vi "wrapandcutimage.vi"(0 "rasterscanned array":sgl[](array[numeric])) -> (1 "imagearray":sgl[][](array[numeric]), 2 "wrap":i32)   [LabVIEW 2015]
panel:
  out "P":dbl
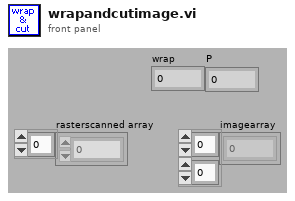
[diagram p1: front panel]
types:
  T1 = typedef "LVRectTypeDef.ctl" = cluster{"Left":i16, "Top":i16, "Right":i16, "Bottom":i16}
  T2 = cluster{"Xpixels":i32, "Vxminref":dbl, "Vxmaxref":dbl, "P":dbl, "Ypixels":i32, "Vyminref":dbl, "Vymaxref":dbl, "srate":sgl, "sAOxy":i32, "timeout":dbl, "type":string, "date":string, "time":string, "Colormap":u16, "Drawing Mode":u16, "Scanning Mode":u16, "square pixels":bool, "square matrix":bool, "Xpixels Img":i32, "Vx-min Img":dbl, "VX-max Img":dbl, "Ypixels Img":i32, "Vy-min Img":dbl, "Vy-max Img ":dbl, "Angle Img":dbl, "autoshutter":bool, "finite":bool, "cont":bool, "wavdet":bool, "measpoints":i32, "avpp":i32, "bufferAO":i32, "bufferAI":i32, "starttick":u32, "waveform":path, "Vx-ref":dbl, "Vy-ref":dbl, "refreshrate":dbl, "refreshbuffer":i32, "tt_cycles":i32, "motorref":refnum<k7>, "mirrorswitch":refnum<k7>, "sample mode":i32, "maxbufferAI":i32, "srateAODO":sgl, "bin":sgl, "Pel":sgl, "Angle draw":dbl, "srate Img":sgl, "ROIimg_plotbounds":T1, "auto OD":bool, "ODfilt":u16, "aAI":i32[], "aCI":i32[], "aAO":u32[], "aDO":u32[], "refwfsize":dbl, "Lifetime":bool, "Vz-Img":dbl, "Vz-ref":dbl, "Vz-reset":dbl, "AIoverride":bool}
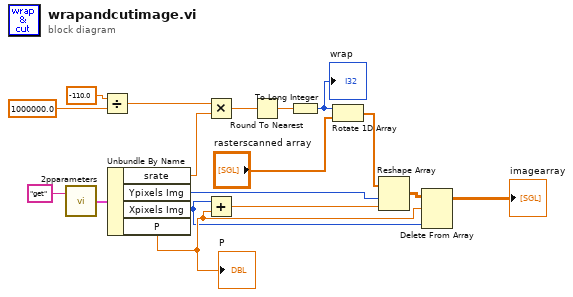
[diagram p0: block diagram]
diagram:
  n1 = call "2pparameters.vi"("command"="get") -> ("params out"=w16:T2)  [unwired: 1 in]
  n2 = Divide(x=-110.0, y=1000000.0) -> (x/y=w11:dbl)
  n3 = Unbundle By Name(w16) -> ("srate"=w10:sgl, "Ypixels Img"=w4:i32, "Xpixels Img"=w2:i32, "P"=w17:dbl)
  "P" <- w17
  n4 = Multiply(x=w11, y=w10) -> (x*y=w5:dbl)
  n5 = Add(x=w2, y=w17) -> (x+y=w3:dbl)
  n6 = Round To Nearest(number=w5) -> (nearest integer value=w9:dbl)
  n7 = To Long Integer(number=w9) -> (32bit integer=w6:i32)
  "wrap" <- w6
  n8 = Rotate 1D Array(1:"rasterscanned array", 2:w6) -> (0:w7:sgl[])
  n9 = Reshape Array(w7, w4, w3) -> (w14:sgl[][])
  n10 = Delete From Array(array=w14, length=w17, index (col)=w2) -> (array with subset deleted=→"imagearray":sgl[][])  [unwired: 1 in, 1 out]
